vi "Global_CMD_ACT_Data In.vi"() -> ()   [LabVIEW 2020, in "Feeder_ACT.lvlib"]
uses:
  roboRIO Code/Systems/Feeder/Feeder_ACT.lvlib
  Cluster_CMD_ACT_Data.ctl
  roboRIO Code/Systems/Feeder/ENUM_CMD Mode.ctl
panel:
  in  "CMD_ACT_Feeder_Data":T1
  # "The Names of the Data items in the Global Variable MUST describe who the Single Writer is\nFor Command Globals the Commander(CMD) represents Teleop or Autonomous or other command loop.\nThe naming convention for a Command Actuator Global is:   \n\nCMD_ACT_SubSystem_Data Name\n\nExample:\nCMD_ACT_Drive_Data\nCMD_ACT_Hopper_Eject Ball"
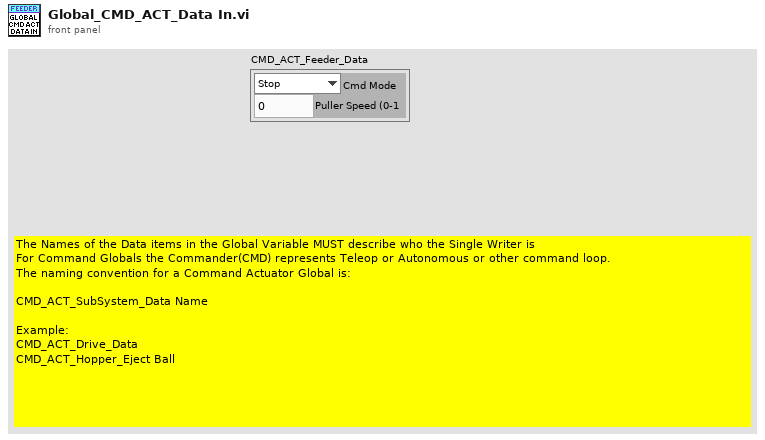
[diagram p1: front panel]
types:
  T1 = typedef "Feeder_ACT.lvlib/Cluster_CMD_ACT_Data.ctl" = cluster{"Cmd Mode":T2, "Puller Speed (0-1":dbl}
  T2 = typedef "Feeder_ACT.lvlib/ENUM_CMD Mode.ctl" = enum16{"Stop", "Feed Pos 1", "Feed Pos 2", "Fead Full", "Back"}
diagram:
